vi "File Page - Init Events.vi"(8 "error in (no error)":errorcluster, 9 "Stop Trig Ref":refnum<k24>, 10 "Start Trig Ref":refnum<k24>, 11 "File Ctl Refs in":T1) -> (0 "error out":errorcluster, 1 "Event Registration Refnum":refnum<event-registration>, 3 "File Ctl Refs out":T1)   [LabVIEW 2015, in "Waveform Data Logger System Explorer.lvlib"]
uses:
  Waveform Data Logger System Explorer.lvlib
  NationalInstruments.VeriStand.SystemStorageUI
  Types/File Ctl Refs.ctl
  Types/File - Spec Ctl Refs.ctl
  Types/File - Wfm Ctl Refs.ctl
  Types/File - Settings Ctl Refs.ctl
  Classes/Log File Specifications/Log File Specification/File Conflict Operation.ctl
  Types/File - Start Trig Ctl Refs.ctl
  Shared/Types/Start Trigger.ctl
  Shared/Types/Default Trigger.ctl
  Shared/Types/Digital Trigger.ctl
  Shared/Types/Analog Trigger.ctl
  Shared/Types/In Range Trigger.ctl
  Shared/Types/Value Change Trigger.ctl
  Shared/Types/Boolean Trigger.ctl
  Types/Single Node Browser Data.ctl
  <vilib>/NI Veristand/UI Controls/Single Node Browser/Single Node Browser Ref.ctl
  <vilib>/NI Veristand/UI Controls/Single Node Browser/Callback Type.ctl
  <vilib>/NI Veristand/UI Controls/Single Node Browser/Net Event Data.ctl
  <vilib>/NI Veristand/UI Controls/Single Node Browser/Net Event.ctl
  Types/File - Stop Trig Ctl Refs.ctl
  Shared/Types/Stop Trigger.ctl
  Types/File - Advanced Ctl Refs.ctl
  Types/Log Timestamps.ctl
  <vilib>/NI Veristand/Custom Device API/Custom Device API.lvlib
  <vilib>/NI Veristand/UI Controls/Single Node Browser/NI_VS UI Single Node Browser.lvlib
  Classes/Log File Specifications/Log File Specification/Log File Specification.lvclass
  Shared/Waveform Data Logger Shared.lvlib
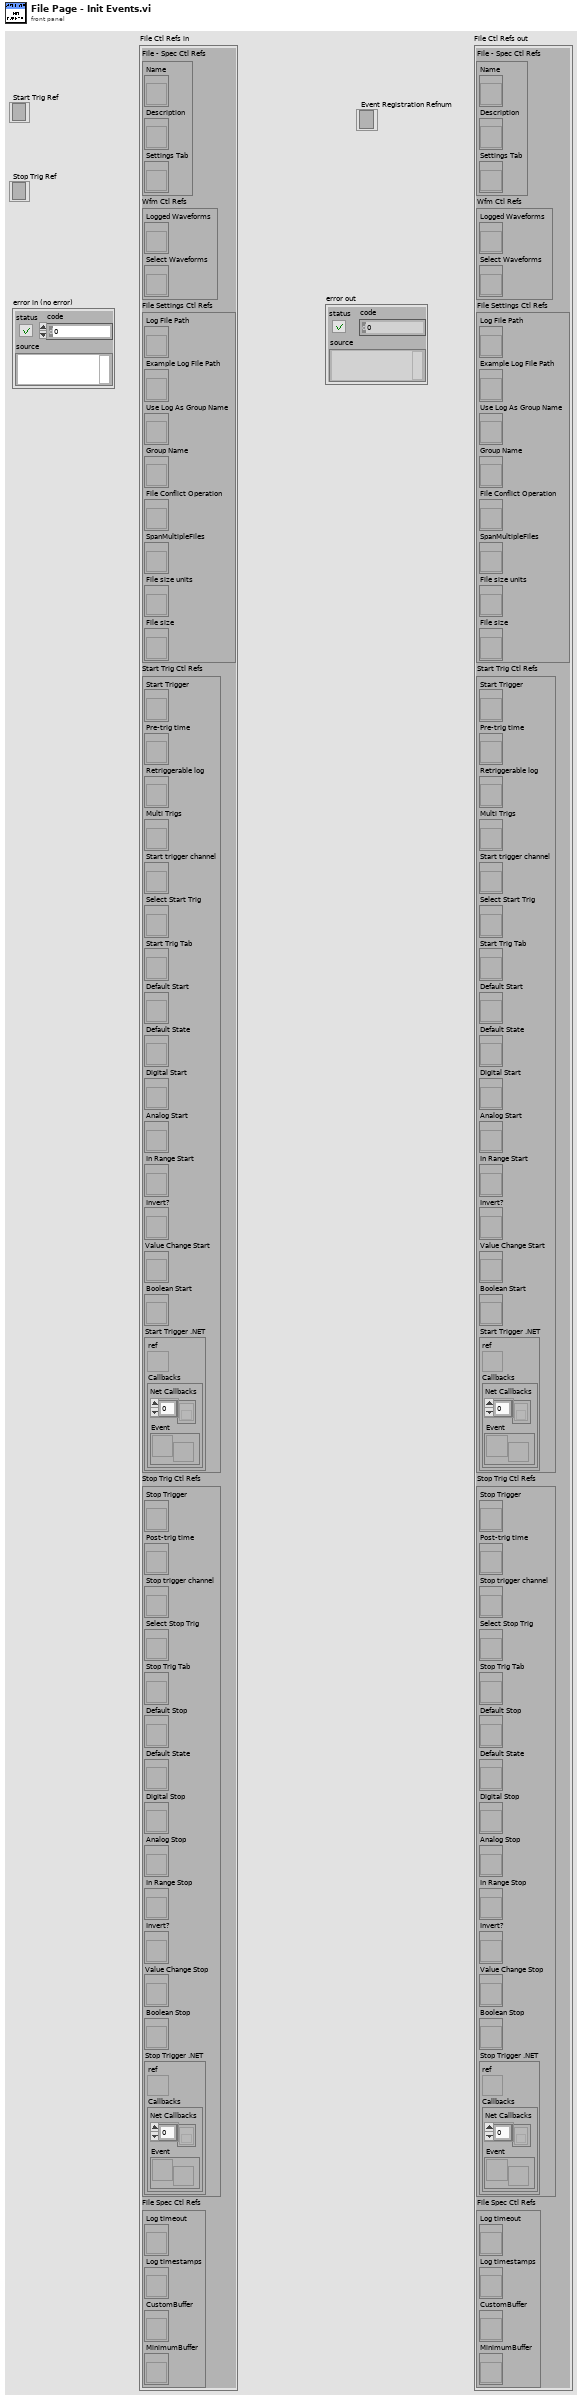
[diagram p1: front panel]
types:
  T1 = typedef "Waveform Data Logger System Explorer.lvlib/File Ctl Refs.ctl" = cluster{"File Spec Ctl Refs":T2, "Wfm Ctl Refs":T3, "File Settings Ctl Refs":T4, "Start Trig Ctl Refs":T5, "Stop Trig Ctl Refs":T9, "File Spec Ctl Refs":T10}
  T2 = typedef "Waveform Data Logger System Explorer.lvlib/File - Spec Ctl Refs.ctl" = cluster{"Name":refnum<vi>, "Description":refnum<vi>, "Settings Tab":refnum<vi>}
  T3 = typedef "Waveform Data Logger System Explorer.lvlib/File - Wfm Ctl Refs.ctl" = cluster{"Logged Waveforms":refnum<vi>, "Select Waveforms":refnum<vi>}
  T4 = typedef "Waveform Data Logger System Explorer.lvlib/File - Settings Ctl Refs.ctl" = cluster{"Log File Path":refnum<vi>, "Example Log File Path":refnum<vi>, "Use Log As Group Name":refnum<vi>, "Group Name":refnum<vi>, "File Conflict Operation":refnum<vi>, "SpanMultipleFiles":refnum<vi>, "File size units":refnum<vi>, "File size":refnum<vi>}
  T5 = typedef "Waveform Data Logger System Explorer.lvlib/File - Start Trig Ctl Refs.ctl" = cluster{"Start Trigger":refnum<vi>, "Pre-trig time":refnum<vi>, "Retriggerable log":refnum<vi>, "Multi Trigs":refnum<vi>, "Start trigger channel":refnum<vi>, "Select Start Trig":refnum<vi>, "Start Trig Tab":refnum<vi>, "Default Start":refnum<vi>, "Default State":refnum<vi>, "Digital Start":refnum<vi>, "Analog Start":refnum<vi>, "In Range Start":refnum<vi>, "Invert?":refnum<vi>, "Value Change Start":refnum<vi>, "Boolean Start":refnum<vi>, "Start Trigger .NET":T6}
  T6 = typedef "Waveform Data Logger System Explorer.lvlib/Single Node Browser Data.ctl" = cluster{"ref":T7, "Callbacks":T8}
  T7 = typedef "NI_VS UI Single Node Browser.lvlib/Single Node Browser Ref.ctl" = refnum<k24>
  T8 = typedef "NI_VS UI Single Node Browser.lvlib/Callback Type.ctl" = cluster{"Net Callbacks":refnum<k27>[], "Event":refnum<user-event>}
  T9 = typedef "Waveform Data Logger System Explorer.lvlib/File - Stop Trig Ctl Refs.ctl" = cluster{"Stop Trigger":refnum<vi>, "Post-trig time":refnum<vi>, "Stop trigger channel":refnum<vi>, "Select Stop Trig":refnum<vi>, "Stop Trig Tab":refnum<vi>, "Default Stop":refnum<vi>, "Default State":refnum<vi>, "Digital Stop":refnum<vi>, "Analog Stop":refnum<vi>, "In Range Stop":refnum<vi>, "Invert?":refnum<vi>, "Value Change Stop":refnum<vi>, "Boolean Stop":refnum<vi>, "Stop Trigger .NET":T6}
  T10 = typedef "Waveform Data Logger System Explorer.lvlib/File - Advanced Ctl Refs.ctl" = cluster{"Log timeout":refnum<vi>, "Log timestamps":refnum<vi>, "CustomBuffer":refnum<vi>, "MinimumBuffer":refnum<vi>}
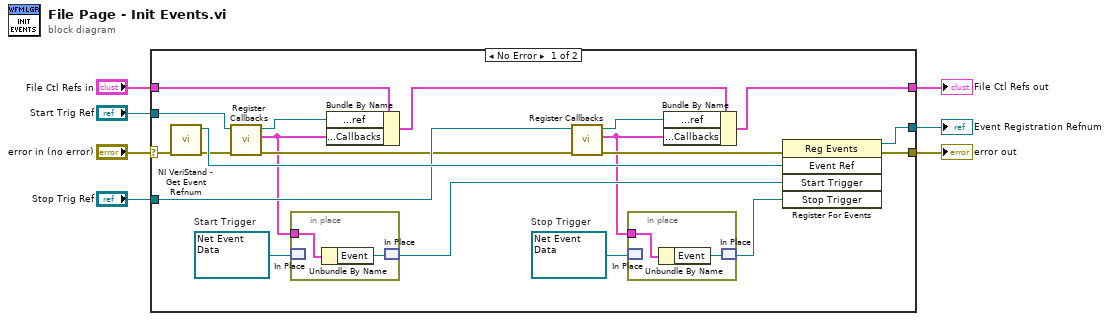
[diagram p0: block diagram]
diagram:
  n1 = case shown="No Error" "error in (no error)" {
    selector: "error in (no error)" -> [w26 w33]
    tunnel: [w21 w33] -> w6
    tunnel: "Stop Trig Ref" -> [w25 _]
    tunnel: "Start Trig Ref" -> [w24 _]
    tunnel: [w20 _] -> w1
    tunnel: [w14 w32] -> w2
    tunnel: "File Ctl Refs in" -> [w16 w32]
    frame No Error {
      w10 = refnum<user-event> refnum  # Stop Trigger
      w13 = refnum<user-event> refnum  # Start Trigger
      n2 = call <vilib>:"NI VeriStand - Get Event Refnum.vi"("error in (no error)"=w26) -> ("error out"=w19:errorcluster, "Event Ref"=w27:refnum<user-event>)  [unwired: 9 out]
      n3 = call <vilib>:"Register Callbacks.vi"("error in (no error)"=w19, "Single Node Browser"=w24) -> ("error out"=w18:errorcluster, "Callbacks"=w12:T8, "Single Node Browser dup"=w23:T7)  [unwired: 7 in]
      n4 = in-place {
        in-place-border: w12 -> [w31]
        n5 = in-place-match #1(w13) -> ()  [unwired: 1 out]
        n6 = Unbundle By Name(w31) -> ("Event"=w30:refnum<user-event>)
        n7 = in-place-match #1(w30) -> (w11:refnum<user-event>)
      }
      n8 = Bundle By Name(cluster=w16, "Start Trig Ctl Refs.Start Trigger .NET.ref"=w23, "Start Trig Ctl Refs.Start Trigger .NET.Callbacks"=w12) -> (w15:T1)
      n9 = call <vilib>:"Register Callbacks.vi"("error in (no error)"=w18, "Single Node Browser"=w25) -> ("error out"=w17:errorcluster, "Callbacks"=w9:T8, "Single Node Browser dup"=w22:T7)  [unwired: 7 in]
      n10 = in-place {
        in-place-border: w9 -> [w29]
        n11 = in-place-match #2(w10) -> ()  [unwired: 1 out]
        n12 = Unbundle By Name(w29) -> ("Event"=w28:refnum<user-event>)
        n13 = in-place-match #2(w28) -> (w8:refnum<user-event>)
      }
      n14 = Bundle By Name(cluster=w15, "Stop Trig Ctl Refs.Stop Trigger .NET.ref"=w22, "Stop Trig Ctl Refs.Stop Trigger .NET.Callbacks"=w9) -> (w14:T1)
      n15 = register-events(error in=w17, w27, w11, w8) -> (reference out=w20:refnum<event-registration>, error out=w21:errorcluster)  [unwired: 1 in]
    }
    frame Error {
    }
  }
  "error out" <- w6
  "File Ctl Refs out" <- w2
  "Event Registration Refnum" <- w1
